vi "convert input indicies to typedef data.vi"(11 "Input Indicies":i32[](array[numeric])) -> (3 "Inputs from system":T1)   [LabVIEW 2013, in "fixed channel tag bus module.lvclass"]
uses:
  fixed channel tag bus module.lvclass
  inputs.ctl
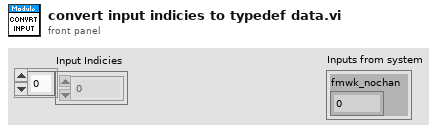
[diagram p1: front panel]
types:
  T1 = typedef "fixed channel tag bus module.lvclass/inputs.ctl" = cluster{"fmwk_nochan":i32}
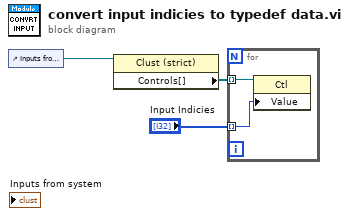
[diagram p0: block diagram]
diagram:
  n1 = control-ref of="Inputs from system"() -> (w3:refnum<vi>)
  n2 = property class="Clust (strict)"(reference=w3) -> ("Controls[]"=w2:refnum<vi>[])  [unwired: 1 in, 2 out]
  n3 = for {
    tunnel: w2 -> [w5] mode=indexing
    tunnel: "Input Indicies" -> [w4] mode=indexing
    n4 = property class="Ctl"(reference=w5, "Value"=w4) -> ()  [unwired: 1 in, 2 out]
  }
